vi "ReleaseSetListPrefNotifier.vi"(2 "error in (no error)":errorcluster, 3 "Preferences in":refnum<class "SetListPrefs.lvclass">) -> (0 "error out":errorcluster, 1 "Preferences out":refnum<class "SetListPrefs.lvclass">)   [LabVIEW 2013, in "SetListPrefs.lvclass"]
uses:
  SetListPrefs.lvclass
  SetListPrefs.lvclass/SetListPrefs.ctl
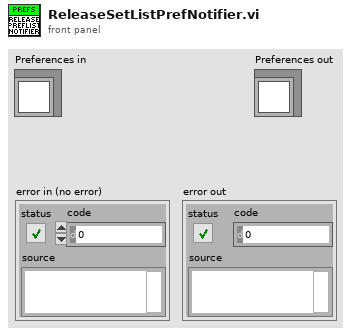
[diagram p1: front panel]
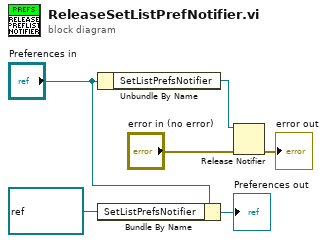
[diagram p0: block diagram]
diagram:
  n1 = Unbundle By Name("Preferences in") -> ("SetListPrefsNotifier"=w1:refnum<notifier>)
  n2 = Bundle By Name(cluster="Preferences in", "SetListPrefsNotifier"=refnum<notifier> refnum) -> (→"Preferences out":refnum<class "SetListPrefs.lvclass">)
  n3 = Release Notifier(notifier=w1, error in (no error)="error in (no error)") -> (error out=→"error out":errorcluster)  [unwired: 1 in, 2 out]
